vi "Reduce Timeout.vi"(8 "error in (no error)":errorcluster, 10 "New Timeout time(ms)":i32, 11 "Response Core in":refnum<class "Response Core.lvclass">) -> (0 "error out":errorcluster, 1 "Timeout time reduced?":bool, 3 "Response Core out":refnum<class "Response Core.lvclass">)   [LabVIEW 2020, in "Publisher.lvlib" / "Response Core.lvclass"]
doc: "Reduce the timeout time on the Response Core if possible."
uses:
  Response Core.lvclass
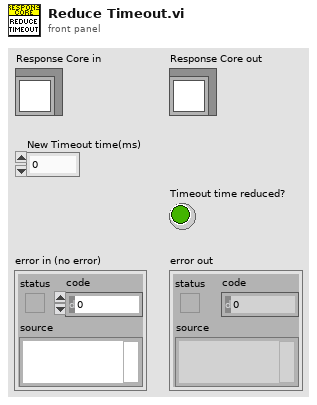
[diagram p1: front panel]
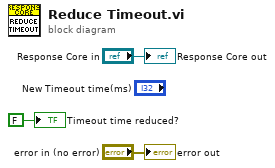
[diagram p0: block diagram]
diagram:
  "error out" <- "error in (no error)"
  "Response Core out" <- "Response Core in"
  "Timeout time reduced?" <- FALSE ("Timeout time reduced?")
